vi "Read Lifetime.vi"(7 "Actor in":refnum<class "Actor.lvclass">) -> (2 "Lifetime":T1)   [LabVIEW 2020, in "jettl.lvlib" / "Actor Specific.lvlib"]
uses:
  Actor Specific.lvlib
  Actor/Actor.lvclass
  Lifetime.ctl
  jettl.lvlib
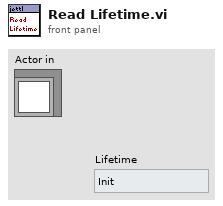
[diagram p1: front panel]
types:
  T1 = typedef "jettl.lvlib/Lifetime.ctl" = enum16{"Init", "Spawn", "Setup", "Teardown Before Running", "Running", "Stop Called", "Stopping With Children", "Stopping Without Children", "Teardown After Running", "Stopped"}
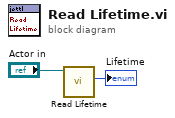
[diagram p0: block diagram]
diagram:
  n1 = call-dynamic "Read Lifetime.vi"("Actor in"="Actor in") -> ("Lifetime"=→"Lifetime":T1)  [unwired: 10 in]
